vi "Digital Read 1 channel.vi"(8 "error in (no error)":errorcluster, 11 "Sensor Channel":i32) -> (0 "error out":errorcluster, 3 "Sensor Value":bool)   [LabVIEW 2016]
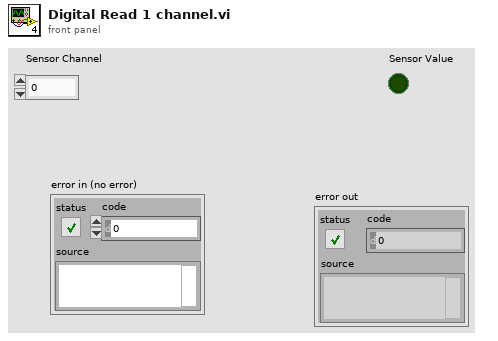
[diagram p1: front panel]
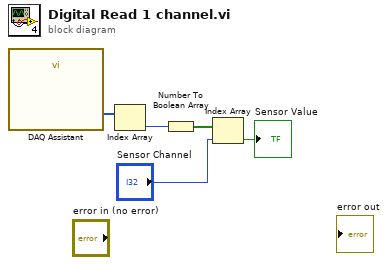
[diagram p0: block diagram]
diagram:
  n1 = call "DAQ Assistant"() -> ("data"=w5:u32[])  [unwired: 17 in, 2 out]
  n2 = Index Array(array=w5) -> (element=w4:u32)  [unwired: 1 in]
  n3 = Number To Boolean Array(number=w4) -> (Boolean array=w2:bool[])
  n4 = Index Array(array=w2, index="Sensor Channel") -> (element=→"Sensor Value":bool)
